vi "Header n Clear Packet.vi"(6 "Hex String in":string, 9 "Stop Single Frquency":bool, 10 "Port Number":i32=2, 11 "FPGA MAC":string) -> (2 "Hex Length":i32, 3 "Hex String out":string)   [LabVIEW 2020]
uses:
  Globals/FPGA Globals.vi
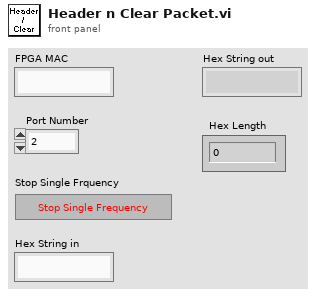
[diagram p1: front panel]
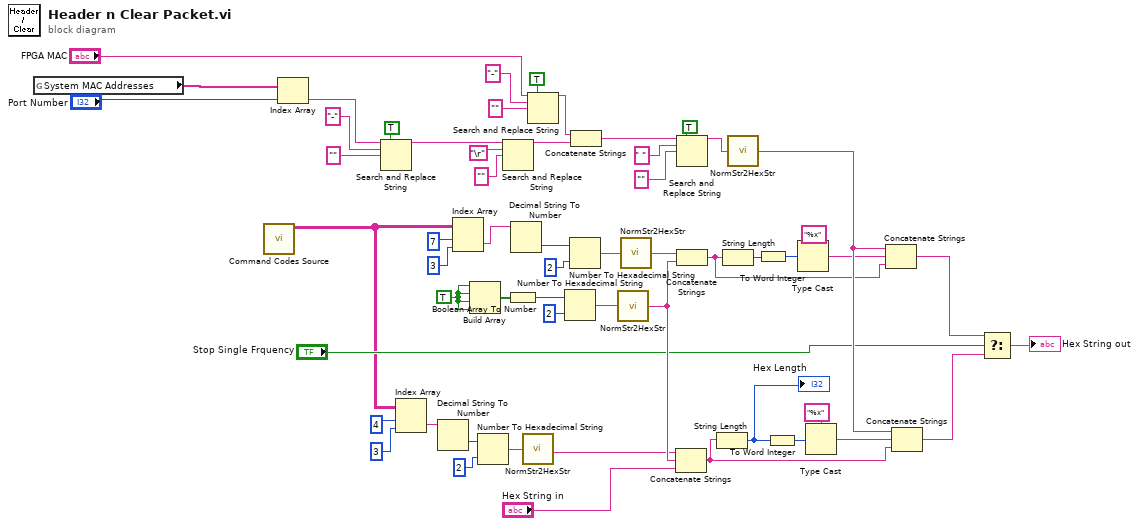
[diagram p0: block diagram]
diagram:
  w43 = TRUE ("replace all? (F)")
  n1 = global read "FPGA Globals.vi" "System MAC Addresses"() -> (w2:string[])
  n2 = call "Command Codes Source.vi"() -> ("Commands for FPGA"=w1:string[][])  [unwired: 11 in]
  n3 = Index Array(array=w2, index="Port Number") -> (element=w9:string)
  n4 = Search and Replace String(replace all?=TRUE ("replace all? (F)"), input string=w9, search string="-", replace string="" ("replace string (\"\")")) -> (result string=w16:string)  [unwired: 4 in, 3 out]
  n5 = Index Array(array=w1, index (row)=4, index (col)=3 ("disabled index (col)")) -> (element=w19:string)
  n6 = Decimal String To Number(string=w19) -> (number=w20:i32)  [unwired: 2 in, 1 out]
  n7 = Index Array(array=w1, index (row)=7, index (col)=3 ("disabled index (col)")) -> (element=w30:string)
  n8 = Build Array(w43, w43, w43, w43) -> (w42:bool[])
  n9 = Number To Hexadecimal String(1:i16 2 ("width (-)"), 2:w20) -> (0:w26:string)
  n10 = Search and Replace String(input string=w16, search string="\r", replace string="" ("replace string (\"\")")) -> (result string=w25:string)  [unwired: 5 in, 3 out]
  n11 = Boolean Array To Number(Boolean array=w42) -> (number=w40:u32)
  n12 = Decimal String To Number(string=w30) -> (number=w29:i32)  [unwired: 2 in, 1 out]
  n13 = call "NormStr2HexStr.vi"("string"=w26) -> ("hex string"=w54:string)
  n14 = Search and Replace String(replace all?=TRUE ("replace all? (F)"), input string="FPGA MAC", search string="-", replace string="" ("replace string (\"\")")) -> (result string=w22:string)  [unwired: 4 in, 3 out]
  n15 = Number To Hexadecimal String(1:i16 2 ("width (-)"), 2:w40) -> (0:w44:string)
  n16 = Number To Hexadecimal String(1:i16 2 ("width (-)"), 2:w29) -> (0:w33:string)
  n17 = Concatenate Strings(w22, w25) -> (w23:string)
  n18 = call "NormStr2HexStr.vi"("string"=w44) -> ("hex string"=w55:string)
  n19 = call "NormStr2HexStr.vi"("string"=w33) -> ("hex string"=w34:string)
  n20 = Concatenate Strings(w54, w55, "Hex String in") -> (w53:string)
  n21 = Search and Replace String(replace all?=TRUE ("replace all? (F)"), input string=w23, search string=" ", replace string="" ("replace string (\"\")")) -> (result string=w27:string)  [unwired: 4 in, 3 out]
  n22 = Concatenate Strings(w34, w55) -> (w38:string)
  n23 = String Length(string=w53) -> (length=w50:i32)
  "Hex Length" <- w50
  n24 = String Length(string=w38) -> (length=w35:i32)
  n25 = call "NormStr2HexStr.vi"("string"=w27) -> ("hex string"=w51:string)
  n26 = To Word Integer(number=w35) -> (16bit integer=w36:i16)
  n27 = To Word Integer(number=w50) -> (16bit integer=w49:i16)
  n28 = Type Cast(type="%x", x=w36) -> (*(type *) &x=w39:string)
  n29 = Type Cast(type="%x", x=w49) -> (*(type *) &x=w52:string)
  n30 = Concatenate Strings(w51, w39, w38) -> (w45:string)
  n31 = Concatenate Strings(w51, w52, w53) -> (w47:string)
  n32 = Select(t=w45, s="Stop Single Frquency", f=w47) -> (s? t:f=→"Hex String out":string)
